vi "Calculate Samples.vi"(8 "error in (no error)":errorcluster, 11 "Ramp Stimulus in":refnum<class "Ramp Stimulus.lvclass">) -> (0 "error out":errorcluster, 3 "Ramp Stimulus out":refnum<class "Ramp Stimulus.lvclass">)   [LabVIEW 2015, in "Ramp Stimulus.lvclass"]
uses:
  Ramp Stimulus.lvclass
  Ramp Stimulus.lvclass/Ramp Stimulus.ctl
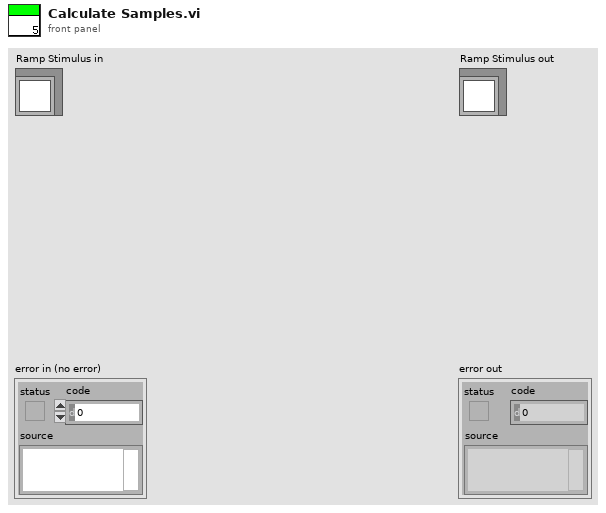
[diagram p1: front panel]
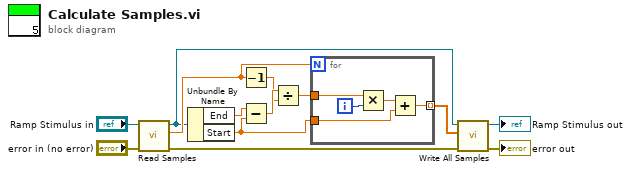
[diagram p0: block diagram]
diagram:
  n1 = call-dynamic "Read Samples.vi"("error in (no error)"="error in (no error)", "Stimulus in"="Ramp Stimulus in") -> ("error out"=w3:errorcluster, "Samples"=w8:dbl, "Stimulus out"=w5:refnum<class "Ramp Stimulus.lvclass">)  [unwired: 7 in]
  n2 = Unbundle By Name(w5) -> ("End"=w11:dbl, "Start"=w9:dbl)
  n3 = Decrement(x=w8) -> (x-1=w7:dbl)
  n4 = Subtract(x=w11, y=w9) -> (x-y=w10:dbl)
  n5 = Divide(x=w10, y=w7) -> (x/y=w6:dbl)
  n6 = for {
    N: w8 -> [_]
    tunnel: w9 -> [w18]
    tunnel: w6 -> [w16]
    tunnel: [w14] -> w4 mode=indexing
    i -> [w17]
    n7 = Multiply(x=w16, y=w17) -> (x*y=w15:dbl)
    n8 = Add(x=w15, y=w18) -> (x+y=w14:dbl)
  }
  n9 = call-dynamic "Write All Samples.vi"("error in (no error)"=w3, "All Samples"=w4, "Stimulus in"=w5) -> ("error out"=→"error out":errorcluster, "Stimulus out"=→"Ramp Stimulus out":refnum<class "Ramp Stimulus.lvclass">)  [unwired: 7 in]
